vi "Cxns-Write Configuration.vi"(0 "Connection File Path":path, 2 "Section":string, 5 "Outputs":string[](array[string]), 9 "Endpoints":string[](array[string]), 11 "error in (no error)":errorcluster) -> (15 "error out":errorcluster)   [LabVIEW 2015]
uses:
  <vilib>/Utility/config.llb/Write Key (String).vi
  <vilib>/Utility/config.llb/NI_LVConfig.lvlib
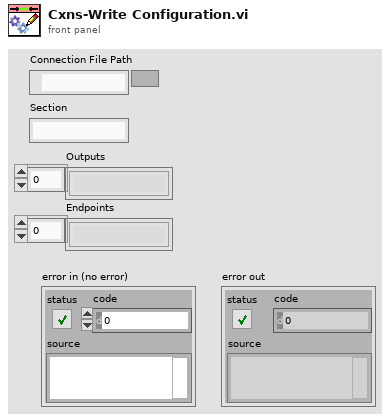
[diagram p1: front panel]
types:
  T1 = typedef "NI_LVConfig.lvlib/Config Data RefNum.ctl" = refnum<k1>
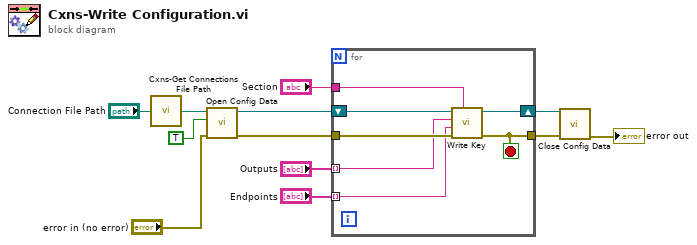
[diagram p0: block diagram]
diagram:
  n1 = call "Cxns-Get Connections File Path.vi"("Connection File Path"="Connection File Path") -> ("Path Out"=w4:path)
  n2 = call <vilib>:"Open Config Data.vi"("error in (no error)"="error in (no error)", "create file if necessary (T)"=TRUE, "configuration file path"=w4) -> ("error out"=w8:errorcluster, "refnum"=w10:T1)  [unwired: 6 in, 1 out]
  n3 = for {
    tunnel: "Outputs" -> [w14] mode=indexing
    tunnel: "Section" -> [w18]
    tunnel: w8 -> [w17]
    tunnel: [w16] -> w7
    shift-right: [w15] -> w6
    shift-left: w10 -> [w19]
    tunnel: "Endpoints" -> [w13] mode=indexing
    stop <- w16 stop-if-true
    n4 = call-poly <vilib>:"Write Key.vi"("section"=w18, "error in (no error)"=w17, "value"=w13, "key"=w14, "refnum"=w19) -> ("error out"=w16:errorcluster, "refnum out"=w15:T1)  [unwired: 4 in, 1 out]
  }
  n5 = call <vilib>:"Close Config Data.vi"("error in (no error)"=w7, "refnum"=w6) -> ("error out"=→"error out":errorcluster)  [unwired: 8 in, 1 out]
